vi "pattern_erstellen.vi"() -> ()   [LabVIEW 2014]
uses:
  <vilib>/userdefined/High Color/IMAQdx.ctl
  <vilib>/vision/driver/NI_Vision_Acquisition_Software.lvlib
  <vilib>/vision/NI_Vision_Development_Module.lvlib
panel:
  in  "Binärbild":bool
  in  "Replace Value":sgl=255.0 format="%.2f"
  in  "Keep/Replace Value (Replace)":bool=TRUE
  in  "Anzahl der Pattern":i32
  in  "Pattern erstellen":bool
  in  "Range":cluster{"Lower value":sgl, "Upper value":sgl}={"Lower value"=128.0, "Upper value"=255.0} {"Upper value" format="%.2f"; "Lower value" format="%.2f"}
  out "Image":T1(plugin-control)
  # "Binäbild einstellungen"
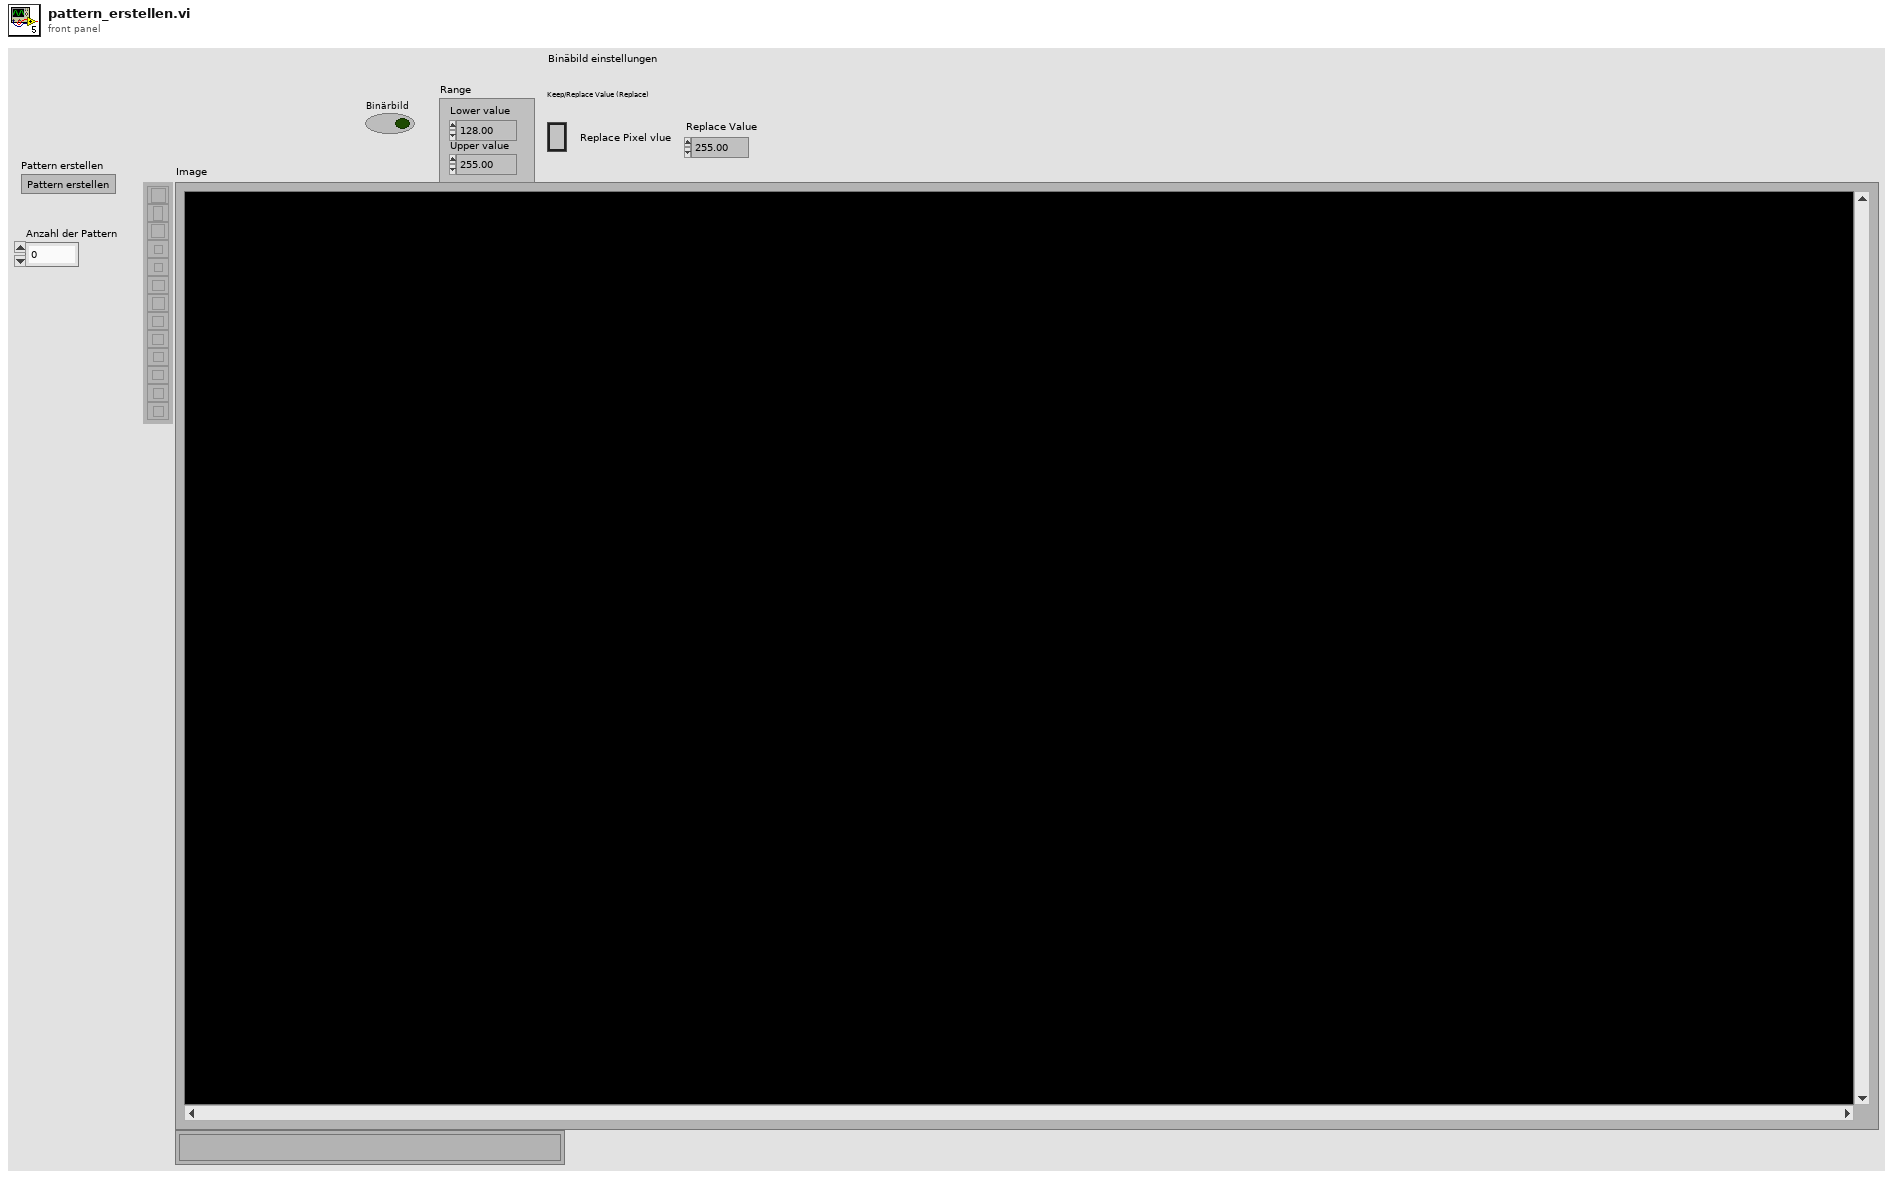
[diagram p1: front panel]
types:
  T1 = typedef "IMAQ Image.ctl" = refnum<image>
  T2 = typedef "Image Type" = u32
  T3 = typedef "IMAQdx.ctl" = refnum<k21>
  T4 = typedef "ROI Descriptor" = cluster{"Global Rectangle":i32[], "Contours":cluster{"ID":enum32{"External", "Internal"}, "Type":u32, "Coordinates":i32[]}[]}
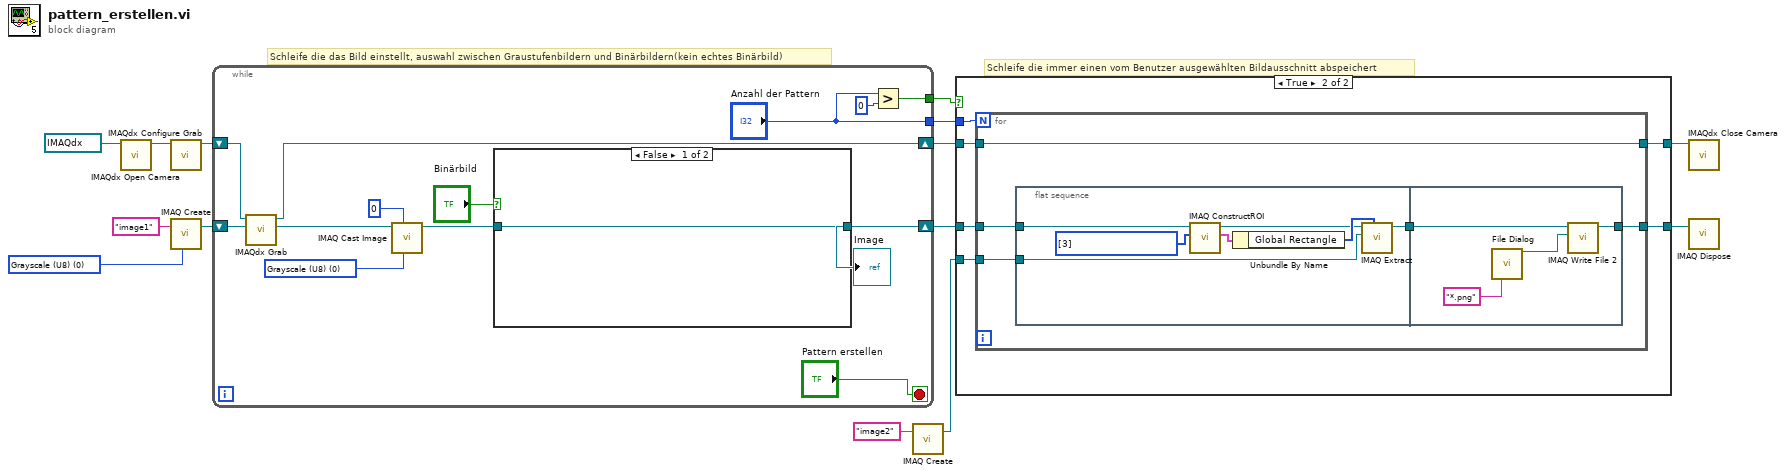
[diagram p0: block diagram]
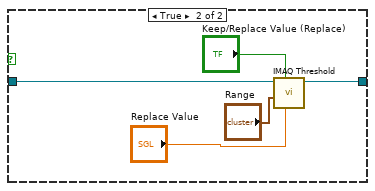
[diagram p3: hidden frame]
diagram:
  w9 = T2 0 items=["Grayscale (U8)", "Grayscale (I16)", "Grayscale (SGL)", "Complex (CSG)", "RGB (U32)", "HSL (U32)", "RGB (U64)", "Grayscale (U16)"] ("Image Type")
  # "Schleife die immer einen vom Benutzer ausgewählten Bildausschnitt abspeichert"
  # "Schleife die das Bild einstellt, auswahl zwischen Graustufenbildern und Binärbildern(kein echtes Binärbild)"
  n1 = call <vilib>:"IMAQdx Open Camera.vi"("Session In"=T3 "cam0") -> ("Session Out"=w14:T3)  [unwired: 9 in, 1 out]
  n2 = call <vilib>:"IMAQdx Configure Grab.vi"("Session In"=w14) -> ("Session Out"=w12:T3)  [unwired: 9 in, 1 out]
  n3 = call "IMAQ Create"("Image Name"="image1", "Image Type"=w9) -> ("New Image"=w11:T1)  [unwired: 3 in, 1 out]
  n4 = while {
    shift-right: [w25] -> w5
    shift-left: w12 -> [w27]
    shift-right: [w19] -> w7
    shift-left: w11 -> [w26]
    tunnel: [w16] -> w2
    tunnel: ["Anzahl der Pattern"] -> w1
    stop <- "Pattern erstellen" stop-if-true
    w24 = T2 0 items=["Grayscale (U8)", "Grayscale (I16)", "Grayscale (SGL)", "Complex (CSG)", "RGB (U32)", "HSL (U32)", "RGB (U64)", "Grayscale (U16)"] ("Image Type")
    n5 = call <vilib>:"IMAQdx Grab.vi"("Image In"=w26, "Session In"=w27) -> ("Image Out"=w22:T1, "Session Out"=w25:T3)  [unwired: 6 in, 2 out]
    n6 = call "IMAQ Cast Image"("Image Type"=w24, "# Shifts"=0, "Image Src"=w22) -> ("Image Dst Out"=w21:T1)  [unwired: 7 in, 1 out]
    n7 = case shown="False" "Binärbild" {
      tunnel: w21 -> [w28 w32]
      tunnel: [w28 w29] -> w19
      frame False {
      }
      frame True {
        n8 = call "IMAQ Threshold"("Replace Value"="Replace Value", "Keep/Replace Value (Replace)"="Keep/Replace Value (Replace)", "Range"="Range", "Image Src"=w32) -> ("Image Dst Out"=w29:T1)  [unwired: 6 in, 1 out]
      }
    }
    "Image" <- w19
    n9 = Greater?(x="Anzahl der Pattern", y=0 ("x")) -> (0:w16:bool)
  }
  n10 = call "IMAQ Create"("Image Name"="image2") -> ("New Image"=w3:T1)  [unwired: 4 in, 1 out]
  n11 = case shown="True" w2 {
    tunnel: w7 -> [w34 w41]
    tunnel: w1 -> [_ w36]
    tunnel: [w35 w40] -> w6
    tunnel: w5 -> [w35 w39]
    tunnel: [w34 w37] -> w4
    tunnel: w3 -> [_ w38]
    frame False {
    }
    frame True {
      n12 = for {
        N: w36 -> [_]
        tunnel: w41 -> [w45]
        tunnel: [w46] -> w40
        tunnel: w39 -> [w46]
        tunnel: w38 -> [w44]
        tunnel: [w42] -> w37
        n13 = flat-sequence {
          tunnel: w45 -> [w50]
          tunnel: w44 -> [w48]
          tunnel: [w47] -> w43
          tunnel: w43 -> [w56]
          tunnel: [w55] -> w42
          frame #0 {
            w53 = u32[] [3] items=["No Selection", "Point", "Line", "Rectangle", "Oval", "Polygon", "Freehand Region", "Annulus", "Zoom", "Pan", "Broken Line", "Freehand Line", "Rotated Rectangle"] ("Tools")
            n14 = call "IMAQ ConstructROI"("Tools"=w53, "Image"=w50) -> ("ROI Descriptor Out"=w51:T4, "Image Out (duplicate)"=w49:T1)  [unwired: 6 in, 2 out]
            n15 = Unbundle By Name(w51) -> ("Global Rectangle"=w52:i32[])
            n16 = call "IMAQ Extract"("Optional Rectangle"=w52, "Image Dst"=w48, "Image Src"=w49) -> ("Image Dst Out"=w47:T1)  [unwired: 7 in, 1 out]
          }
          frame #1 {
            n17 = call "File Dialog"("pattern (all files)"="*.png" ("prompt")) -> ("selected path"=w57:path)  [unwired: 11 in, 3 out]
            n18 = call-poly "IMAQ Write File 2"("File Path"=w57, "Image"=w56) -> ("Image Out (duplicate)"=w55:T1)  [unwired: 8 in, 1 out]
          }
        }
      }
    }
  }
  n19 = call <vilib>:"IMAQdx Close Camera.vi"("Session In"=w6) -> ()  [unwired: 10 in, 1 out]
  n20 = call "IMAQ Dispose"("Image"=w4) -> ()  [unwired: 5 in, 1 out]
